vi "Construct Sequence.vi"(8 "error in":errorcluster, 11 "Cal Sequence Builder in":refnum<class "Cal Sequence Builder.lvclass">) -> (0 "error out":errorcluster, 2 "New Sequence":refnum<class "SEQ.lvclass">, 3 "Cal Sequence Builder out":refnum<class "Cal Sequence Builder.lvclass">)   [LabVIEW 2015, in "Cal Sequence Builder.lvclass"]
doc: "Construct an O3 calibration sequence based on user input provided through Config Data. Config Data is ordered as follows:\n* Purge volume time\n* Zero check time\n* Flow rates (array of singles) - these are actually percentages of the FS value recored in the Set O2 to max.\n* O3 stability parameters - cluser of allowable error and # of observations\n* Laser stability parameters - same as previous\n* PAS State DVR - cPAS Data type\n* Number of collected data points during collection step - U16\n* Cell associations - these go PAS-CRDS and are based on the wavelength\n* CRD State DVR - cCRDS Data type"
uses:
  Cal Sequence Builder.lvclass
  Reusable/Sequence/SEQ/SEQ.lvclass
  Change O2 Valve.lvclass
  Set QO2/Set QO2.lvclass
  Get Max Orf Flow/Get Max Orifice Flow.lvclass
  Change Spk Pos/Change Speaker Position.lvclass
  O3 Generator State/Change O3 Generator State.lvclass
  Wait/Wait.lvclass
  Reusable/Data/Double/Double.lvclass
  config data.ctl
  O3 Add Valve/Ozone Addition Valve.lvclass
  Reusable/Data/Boolean/Boolean Data.lvclass
  Change Filter State/Change Filter Position.lvclass
  Get Max Orf Flow/Get Max Orifice Flow.lvclass/Get Max Orifice Flow.ctl
  Reusable/Sequence/Sequence Factory/Sequence Builder.lvclass/Sequence Builder.ctl
  Reusable/Data/Boolean/Boolean Data.lvclass/Boolean Data.ctl
  Wait/Wait.lvclass/Wait.ctl
  Reusable/Sequence/STEPS/LEAVES/Double/Switch DBL.lvclass/Switch DBL.ctl
  Reusable/Sequence/STEPS/LEAVES/Double/Write val.vi
  Get Max Orf Flow/Write Max Qorf DVR.vi
  Reusable/Sequence/Sequence Factory/Accessors/Read Config Data.vi
  Reusable/Data/Data.lvclass
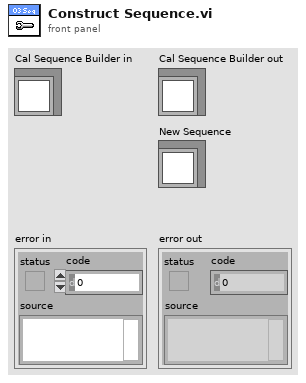
[diagram p1: front panel]
types:
  T1 = typedef "Cal Sequence Builder.lvclass/config data.ctl" = enum16{"purge time", "zero time", "qo2", "o3 stability", "laser stability", "pas state dvr", "collection observations", "associated cells", "crds state dvr", "Init Filter State"}
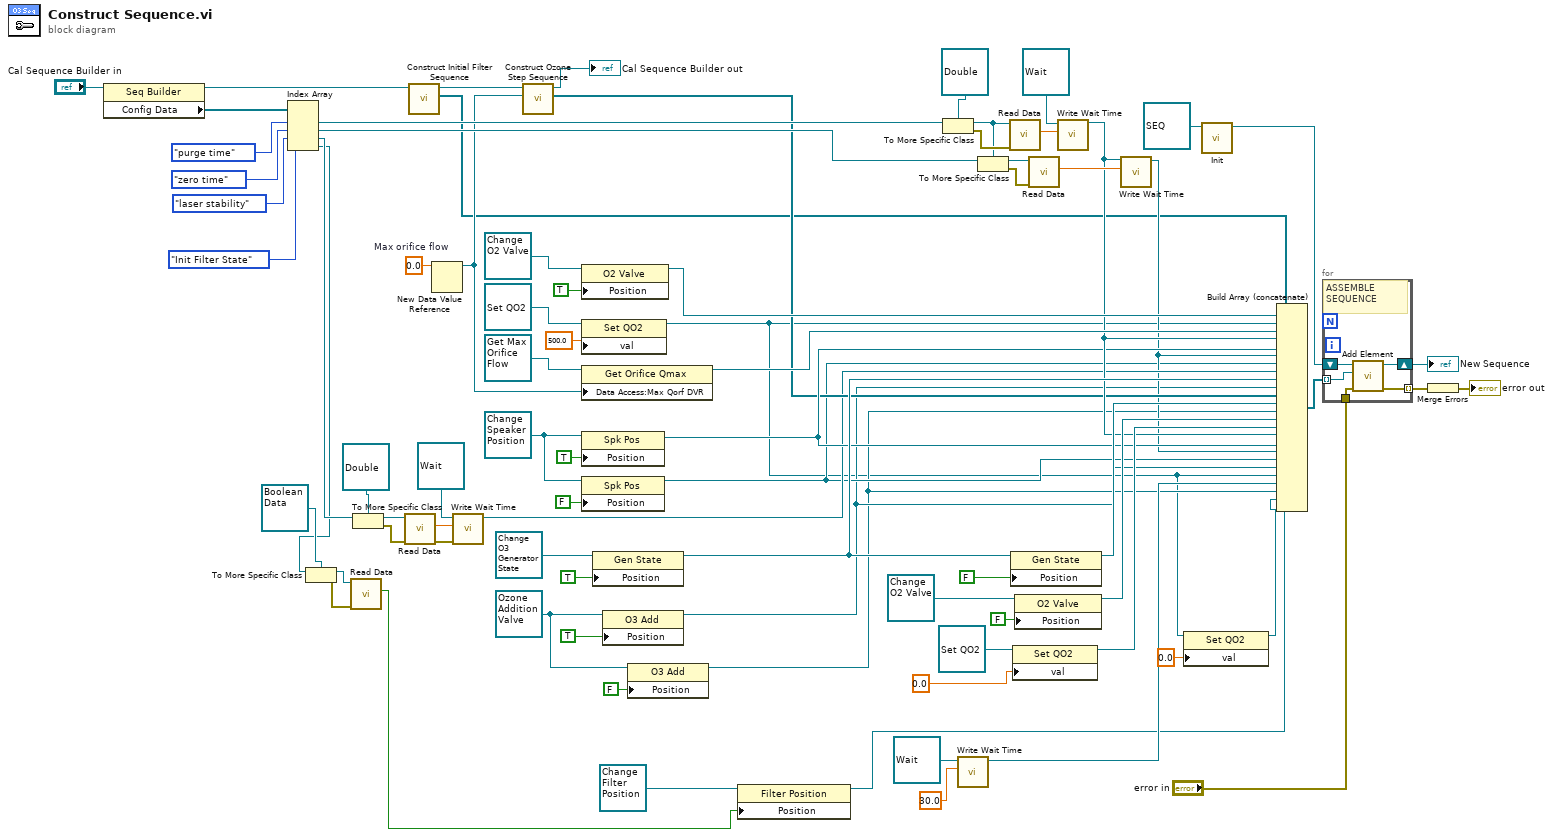
[diagram p0: block diagram]
diagram:
  w23 = refnum<class "Ozone Addition Valve.lvclass"> refnum ("O3 Add")
  w57 = 0.0  # Max orifice flow
  w69 = refnum<class "Change Speaker Position.lvclass"> refnum ("Change Speaker Position.lvclass")
  n1 = property class="Seq Builder"(reference="Cal Sequence Builder in") -> (reference out=w11:refnum<class "Cal Sequence Builder.lvclass">, "Config Data"=w73:refnum<class "Data.lvclass">[])  [unwired: 1 in, 1 out]
  n2 = Index Array(array=w73, index #1=config_data."purge time" ("config data"), index #2=config_data."zero time" ("config data"), index #3=config_data."laser stability" ("config data"), index #4=config_data."Init Filter State" ("config data")) -> (element #1=w65:refnum<class "Data.lvclass">, element #2=w61:refnum<class "Data.lvclass">, element #3=w31:refnum<class "Data.lvclass">, element #4=w6:refnum<class "Data.lvclass">)
  n3 = To More Specific Class(target class=refnum<class "Boolean Data.lvclass"> refnum ("Boolean Data.lvclass"), reference=w6) -> (specific class reference=w5:refnum<class "Boolean Data.lvclass">, error out=w4:errorcluster)  [unwired: 1 in]
  n4 = call "Read Data.vi"("error in (no error)"=w4, "Boolean Data in"=w5) -> ("Data"=w2:bool)  [unwired: 7 in, 2 out]
  n5 = To More Specific Class(target class=refnum<class "Double.lvclass"> refnum ("Base Data Class.lvlib:Double.lvclass"), reference=w31) -> (specific class reference=w32:refnum<class "Double.lvclass">, error out=w26:errorcluster)  [unwired: 1 in]
  n6 = call "Read Data.vi"("error in (no error)"=w26, "Double in"=w32) -> ("error out"=w25:errorcluster, "Data"=w34:dbl)  [unwired: 7 in, 1 out]
  n7 = call "Construct Initial Filter Sequence.vi"("Seq Builder in"=w11) -> ("Init Filter"=w9:refnum<class "STEP.lvclass">[], "Seq Builder out"=w10:refnum<class "Cal Sequence Builder.lvclass">)  [unwired: 8 in, 1 out]
  n8 = New Data Value Reference(data value=w57) -> (data value reference=w36:refnum<data-value>)  [unwired: 1 in, 1 out]
  n9 = call "Write Wait Time.vi"("error in (no error)"=w25, "Wait Time"=w34, "Wait in"=refnum<class "Wait.lvclass"> refnum ("Wait")) -> ("Wait out"=w30:refnum<class "Wait.lvclass">)  [unwired: 7 in, 1 out]
  n10 = call "Construct Ozone Step Sequence.vi"("QO2 DVR"=w36, "Seq Builder in"=w10) -> ("Steps"=w37:refnum<class "STEP.lvclass">[], "Seq Builder out"=→"Cal Sequence Builder out":refnum<class "Cal Sequence Builder.lvclass">)  [unwired: 7 in, 1 out]
  n11 = property class="O2 Valve"(reference=refnum<class "Change O2 Valve.lvclass"> refnum ("O2 Valve"), "Position"=TRUE) -> (reference out=w72:refnum<class "Change O2 Valve.lvclass">)  [unwired: 1 in, 1 out]
  n12 = property class="Set QO2"(reference=refnum<class "Set QO2.lvclass"> refnum ("Set QO2.lvclass"), "val"=500.0) -> (reference out=w14:refnum<class "Set QO2.lvclass">)  [unwired: 1 in, 1 out]
  n13 = property class="Get Orifice Qmax"(reference=refnum<class "Get Max Orifice Flow.lvclass"> refnum ("Get Orifice Qmax"), "Data Access:Max Qorf DVR"=w36) -> (reference out=w56:refnum<class "Get Max Orifice Flow.lvclass">)  [unwired: 1 in, 1 out]
  n14 = property class="Spk Pos"(reference=w69, "Position"=TRUE) -> (reference out=w44:refnum<class "Change Speaker Position.lvclass">)  [unwired: 1 in, 1 out]
  n15 = property class="Spk Pos"(reference=w69, "Position"=FALSE) -> (reference out=w20:refnum<class "Change Speaker Position.lvclass">)  [unwired: 1 in, 1 out]
  n16 = property class="Gen State"(reference=refnum<class "Change O3 Generator State.lvclass"> refnum ("Change O3 Generator State"), "Position"=TRUE) -> (reference out=w54:refnum<class "Change O3 Generator State.lvclass">)  [unwired: 1 in, 1 out]
  n17 = property class="O3 Add"(reference=w23, "Position"=TRUE) -> (reference out=w16:refnum<class "Ozone Addition Valve.lvclass">)  [unwired: 1 in, 1 out]
  n18 = property class="O3 Add"(reference=w23, "Position"=FALSE) -> (reference out=w15:refnum<class "Ozone Addition Valve.lvclass">)  [unwired: 1 in, 1 out]
  n19 = property class="Filter Position"(reference=refnum<class "Change Filter Position.lvclass"> refnum ("Filter Position"), "Position"=w2) -> (reference out=w1:refnum<class "Change Filter Position.lvclass">)  [unwired: 1 in, 1 out]
  n20 = To More Specific Class(target class=refnum<class "Double.lvclass"> refnum ("Base Data Class.lvlib:Double.lvclass"), reference=w65) -> (specific class reference=w55:refnum<class "Double.lvclass">, error out=w63:errorcluster)  [unwired: 1 in]
  n21 = call "Write Wait Time.vi"("Wait Time"=30.0, "Wait in"=refnum<class "Wait.lvclass"> refnum ("Wait")) -> ("Wait out"=w17:refnum<class "Wait.lvclass">)  [unwired: 8 in, 1 out]
  n22 = To More Specific Class(target class=w55, reference=w61) -> (specific class reference=w60:refnum<class "Double.lvclass">, error out=w42:errorcluster)  [unwired: 1 in]
  n23 = call "Read Data.vi"("error in (no error)"=w63, "Double in"=w55) -> ("Data"=w62:dbl)  [unwired: 7 in, 2 out]
  n24 = property class="Gen State"(reference=w54, "Position"=FALSE) -> (reference out=w52:refnum<class "Change O3 Generator State.lvclass">)  [unwired: 1 in, 1 out]
  n25 = property class="Set QO2"(reference=refnum<class "Set QO2.lvclass"> refnum ("Set QO2.lvclass"), "val"=0.0) -> (reference out=w46:refnum<class "Set QO2.lvclass">)  [unwired: 1 in, 1 out]
  n26 = property class="O2 Valve"(reference=refnum<class "Change O2 Valve.lvclass"> refnum ("O2 Valve"), "Position"=FALSE) -> (reference out=w49:refnum<class "Change O2 Valve.lvclass">)  [unwired: 1 in, 1 out]
  n27 = call "Read Data.vi"("error in (no error)"=w42, "Double in"=w60) -> ("Data"=w59:dbl)  [unwired: 7 in, 2 out]
  n28 = call "Write Wait Time.vi"("Wait Time"=w62, "Wait in"=refnum<class "Wait.lvclass"> refnum ("Wait")) -> ("Wait out"=w45:refnum<class "Wait.lvclass">)  [unwired: 8 in, 1 out]
  n29 = call "Write Wait Time.vi"("Wait Time"=w59, "Wait in"=w45) -> ("Wait out"=w21:refnum<class "Wait.lvclass">)  [unwired: 8 in, 1 out]
  n30 = property class="Set QO2"(reference=w14, "val"=0.0) -> (reference out=w12:refnum<class "Set QO2.lvclass">)  [unwired: 1 in, 1 out]
  n31 = call-dynamic "Init.vi"("SEQ in"=refnum<class "SEQ.lvclass"> refnum) -> ("SEQ out"=w80:refnum<class "SEQ.lvclass">)  [unwired: 9 in, 1 out]
  n32 = Build Array (concatenate)(w9, w72, w14, w56, w45, w44, w21, w20, w30, w54, w16, w37, w52, w15, w49, w46, w45, w44, w21, w20, w16, w14, w17, w15, w12, w1) -> (w43:refnum<class "STEP.lvclass">[])
  n33 = for {
    shift-right: [w85] -> w79
    shift-left: w80 -> [w86]
    tunnel: w43 -> [w84] mode=indexing
    tunnel: "error in" -> [w83]
    tunnel: [w82] -> w40 mode=indexing
    # "ASSEMBLE SEQUENCE"
    n34 = call "Add Element.vi"("error in"=w83, "STEP"=w84, "SEQ in"=w86) -> ("error out"=w82:errorcluster, "SEQ out"=w85:refnum<class "SEQ.lvclass">)  [unwired: 7 in]
  }
  "New Sequence" <- w79
  n35 = Merge Errors(w40) -> (→"error out":errorcluster)
